vi "Write Header.vi"(8 "error in (no error)":errorcluster, 11 "Log in":refnum<class "Log.lvclass">) -> (0 "error out":errorcluster)   [LabVIEW 2020, in "Log.lvclass"]
doc: "Writes the Header string to the configured file path.\n\nIf the file already exists, the header is appended rather than the file being overwritten."
uses:
  Log.lvclass
  Log.lvclass/Log.ctl
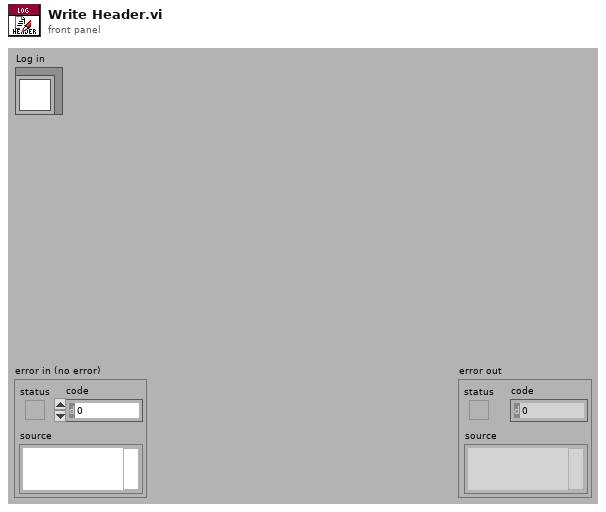
[diagram p1: front panel]
types:
  T1 = enum16{"open", "replace", "create", "open or create", "replace or create", "replace or create with confirmation"}
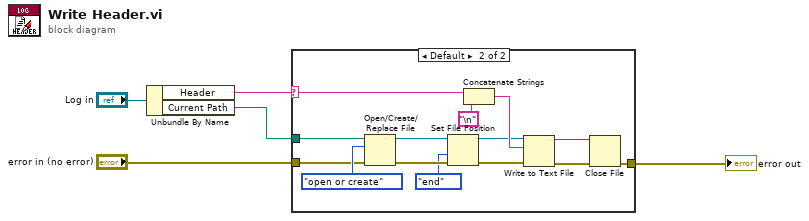
[diagram p0: block diagram]
diagram:
  n1 = Unbundle By Name("Log in") -> ("Header"=w1:string, "Current Path"=w2:path)
  n2 = case shown="Default" w1 {
    selector: w1 -> [_ w9]
    tunnel: w2 -> [_ w10]
    tunnel: "error in (no error)" -> [w6 w8]
    tunnel: [w6 w7] -> w4
    frame "" {
      # "Do not write header if empty. Writing the header also writes a blank line after it which is not desirable if the header is blank."
    }
    frame Default {
      n3 = Open/Create/Replace File(file path (use dialog)=w10, error in=w8, operation (0:open)=T1."open or create") -> (refnum out=w11:refnum<file>, error out=w17:errorcluster)  [unwired: 4 out]
      n4 = Set File Position(refnum=w11, from (0:start)=enum16{"start", "end", "current"}."end", error in=w17) -> (refnum out=w13:refnum<file>, error out=w18:errorcluster)  [unwired: 1 out]
      n5 = Concatenate Strings(w9, "\n") -> (w15:string)
      n6 = Write to Text File(file (use dialog)=w13, text=w15, error in=w18) -> (refnum out=w16:refnum<file>, error out=w19:errorcluster)  [unwired: 2 out]
      n7 = Close File(refnum=w16, error in=w19) -> (error out=w7:errorcluster)  [unwired: 1 out]
    }
  }
  "error out" <- w4
